vi "Filter Get Threshold.vi"(8 "error in (no error)":errorcluster, 11 "threshold":sgl) -> (0 "error out":errorcluster, 2 "function return":u32, 3 "threshold out":sgl)   [LabVIEW 2014, in "atmcd32d.lvlib"]
doc: "unsigned int WINAPI Filter_GetThreshold(float * threshold);"
uses:
  atmcd32d.lvlib
  atmcd32d.dll
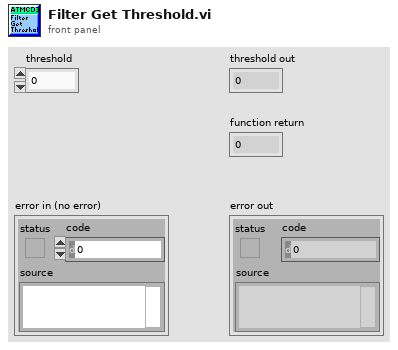
[diagram p1: front panel]
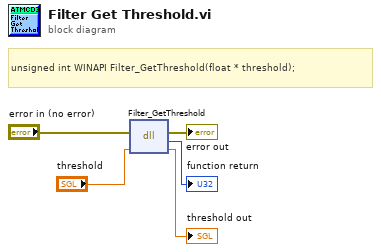
[diagram p0: block diagram]
diagram:
  # "unsigned int WINAPI Filter_GetThreshold(float * threshold);"
  n1 = dll-call lib="C:/Users/Bakir/Documents/Lambda2-Testing/lib/Andorlib/atmcd32d.*" fn="Filter_GetThreshold"(error in="error in (no error)", "threshold"="threshold") -> (error out=→"error out":errorcluster, →"function return":u32, "threshold"=→"threshold out":sgl)  [unwired: 2 in, 1 out]
